vi "GenerateSin.vi"(8 "error in (no error)":errorcluster, 11 "Nested in":refnum<class "Nested.lvclass">) -> (0 "error out":errorcluster, 3 "Nested out":refnum<class "Nested.lvclass">)   [LabVIEW 2020, in "Nested.lvlib" / "Nested.lvclass"]
uses:
  Nested.lvclass
  Nested.lvclass/Nested.ctl
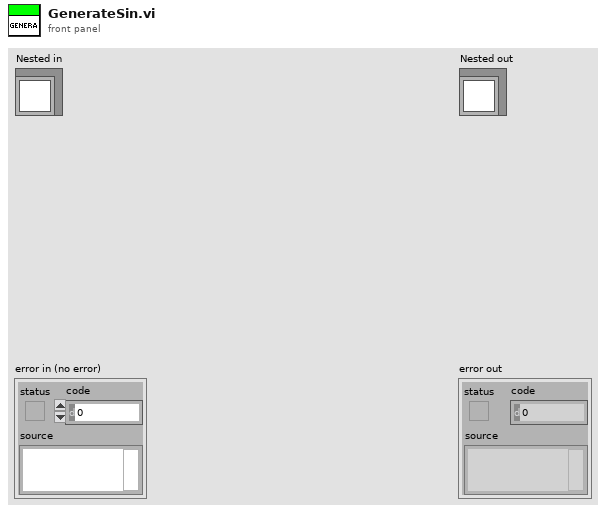
[diagram p1: front panel]
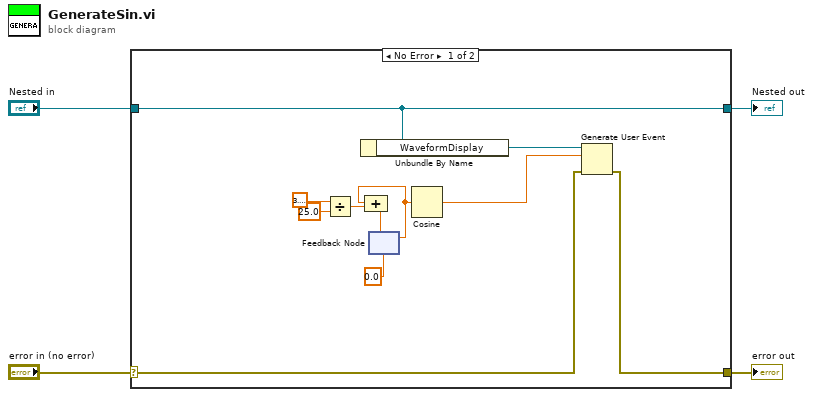
[diagram p0: block diagram]
diagram:
  n1 = case shown="No Error" "error in (no error)" {
    selector: "error in (no error)" -> [w6 w17]
    tunnel: [w5 w17] -> w3
    tunnel: [w9 w16] -> w1
    tunnel: "Nested in" -> [w9 w16]
    frame No Error {
      n2 = Divide(x=3.141592653589793, y=25.0) -> (x/y=w13:dbl)
      n3 = Unbundle By Name(w9) -> ("WaveformDisplay"=w8:refnum<user-event>)
      n4 = feedback #1(0.0) -> (w11:dbl)
      n5 = Compound Arithmetic op=ADD(w11, w13) -> (w12:dbl)
      n6 = feedback-in #1(w12) -> ()
      n7 = Cosine(x=w11) -> (cos(x)=w7:dbl)
      n8 = Generate User Event(user event=w8, event data cluster=w7, error in=w6) -> (error out=w5:errorcluster)  [unwired: 1 in, 1 out]
    }
    frame Error {
    }
  }
  "error out" <- w3
  "Nested out" <- w1
